vi "Path.vi"() -> (3 "All Files in Dir":path[](array[path]))   [LabVIEW 2020]
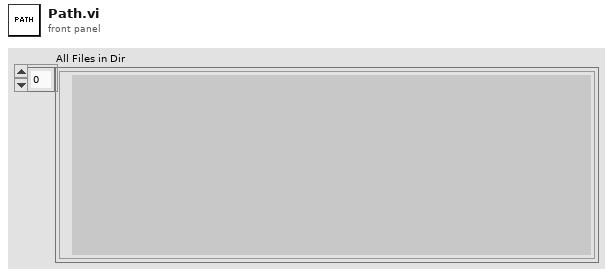
[diagram p1: front panel]
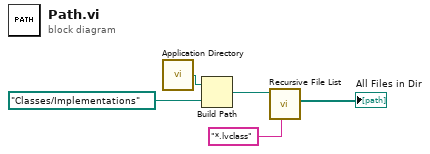
[diagram p0: block diagram]
diagram:
  n1 = call <vilib>:"Application Directory.vi"() -> ("Application Directory"=w2:path)
  n2 = Build Path(base path=w2, name or relative path=path "Classes/Implementations") -> (appended path=w4:path)
  n3 = call <vilib>:"Recursive File List.vi"("pattern"="*.lvclass", "Folder Path"=w4) -> ("All Files in Dir"=→"All Files in Dir":path[])  [unwired: 5 in, 4 out]
